vi "Write I2C.vi"(5 "Address":u8, 6 "NoStop (F)":bool, 7 "Bus":u8, 8 "error in (no error)":errorcluster, 10 "Data":string, 11 "VISA resource name in":refnum<visa-resource-name>) -> (0 "error out":errorcluster, 3 "VISA resource name":refnum<visa-resource-name>)   [LabVIEW 2024, in "CTIPicoVISA.lvlib"]
uses:
  CTIPicoVISA.lvlib
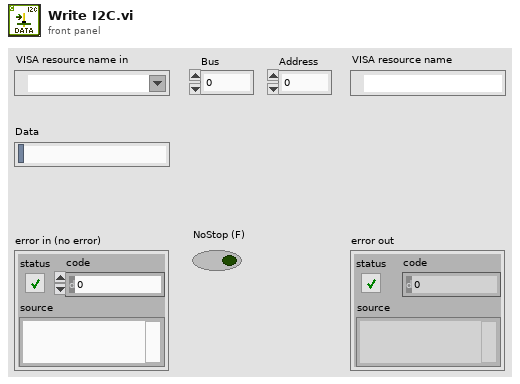
[diagram p1: front panel]
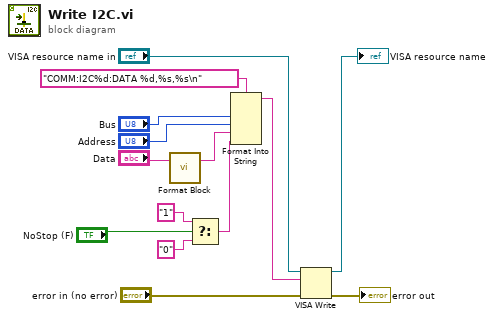
[diagram p0: block diagram]
diagram:
  n1 = call "Format Block.vi"("Data Block"="Data") -> ("Formatted Block"=w1:string)  [unwired: 6 in]
  n2 = Select(t="1", s="NoStop (F)", f="0") -> (s? t:f=w3:string)
  n3 = Format Into String(format string="COMM:I2C%d:DATA %d,%s,%s\n", "Bus", "Address", w1, w3) -> (resulting string=w11:string)  [unwired: 2 in, 1 out]
  n4 = VISA Write(VISA resource name="VISA resource name in", write buffer=w11, error in (no error)="error in (no error)") -> (VISA resource name out=→"VISA resource name":refnum<visa-resource-name>, error out=→"error out":errorcluster)  [unwired: 1 out]
